vi "Initialize Kinect - Copy.vi"() -> (0 "error out":errorcluster, 3 "Reference Out":T1)   [LabVIEW 2011]
uses:
  <vilib>/vision/Image Controls.llb/IMAQ Image.ctl
  Microsoft.Research.Kinect
panel:
  in  "Buffer Size":i32=1
  in  "error in (no error)":errorcluster
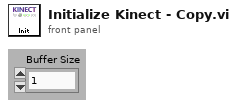
[diagram p1: front panel]
types:
  T1 = cluster{cluster{"queue out":refnum<queue>, "queue out":refnum<queue>}, cluster{"new reference":refnum<k24>, "DepthStream":refnum<k24>, "VideoStream":refnum<k24>, "Event Callback":refnum<k27>, "Event Callback":refnum<k27>}}
  T2 = typedef "IMAQ Image.ctl" = refnum<image>
  T3 = cluster{"queue out":refnum<queue>, "queue out":refnum<queue>}
  T4 = cluster{"new reference":refnum<k24>, "DepthStream":refnum<k24>, "VideoStream":refnum<k24>, refnum<k27>, refnum<k27>}
  T5 = cluster{cluster{"queue out":refnum<queue>, "queue out":refnum<queue>}, cluster{"new reference":refnum<k24>, "DepthStream":refnum<k24>, "VideoStream":refnum<k24>, refnum<k27>, refnum<k27>}}
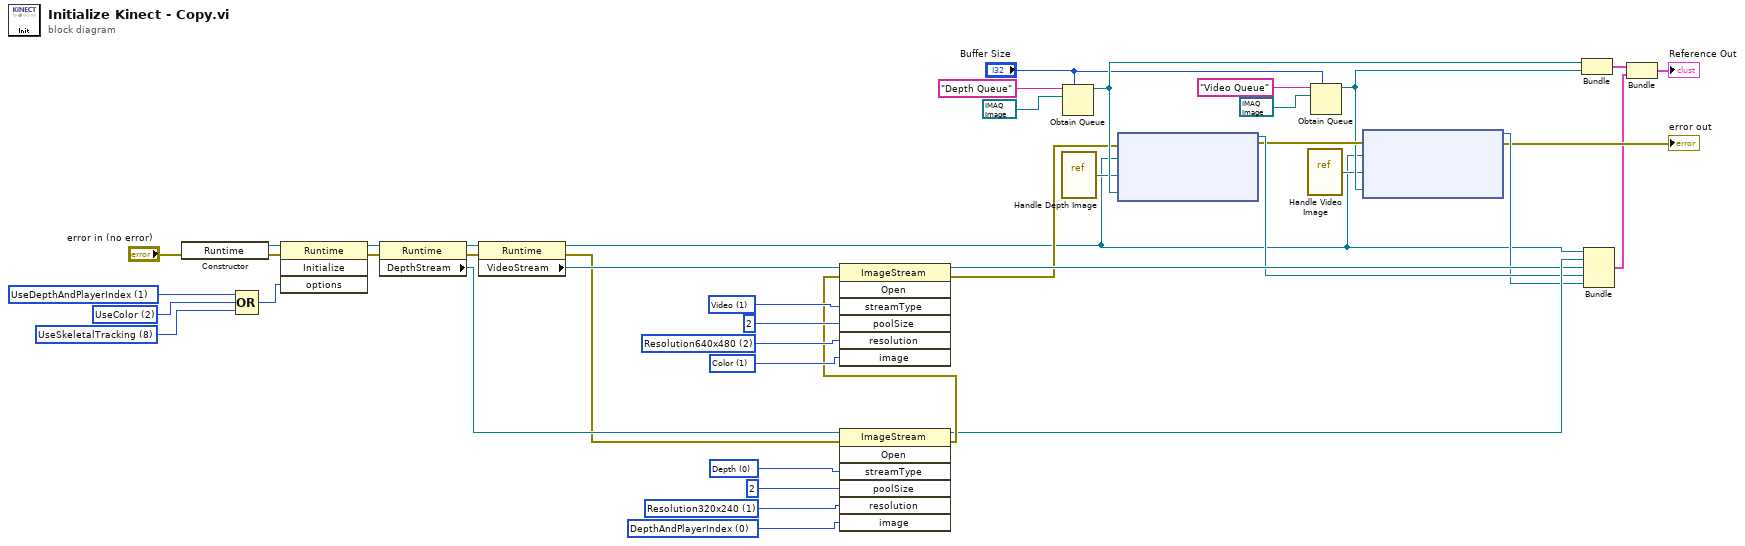
[diagram p0: block diagram]
diagram:
  w25 = 8 items=["UseDepthAndPlayerIndex"=1, "UseColor"=2, "UseSkeletalTracking"=8, "UseDepth"=32] ("options")
  w26 = 2 items=["UseDepthAndPlayerIndex"=1, "UseColor"=2, "UseSkeletalTracking"=8, "UseDepth"=32] ("options")
  w36 = 1 items=["Resolution80x60"=0, "Resolution320x240"=1, "Resolution640x480"=2, "Resolution1280x1024"=3, "Invalid"=-1] ("resolution")
  w27 = 1 items=["UseDepthAndPlayerIndex"=1, "UseColor"=2, "UseSkeletalTracking"=8, "UseDepth"=32] ("options")
  w39 = 0 items=["DepthAndPlayerIndex", "Color", "ColorYuv", "ColorYuvRaw", "Depth", "DepthAndPlayerIndexInColorSpace", "DepthInColorSpace", "ColorInDepthSpace"] ("image")
  w31 = 1 items=["DepthAndPlayerIndex", "Color", "ColorYuv", "ColorYuvRaw", "Depth", "DepthAndPlayerIndexInColorSpace", "DepthInColorSpace", "ColorInDepthSpace"] ("image")
  w32 = 2 items=["Resolution80x60"=0, "Resolution320x240"=1, "Resolution640x480"=2, "Resolution1280x1024"=3, "Invalid"=-1] ("resolution")
  w34 = 1 items=["Depth"=0, "Video"=1, "Invalid"=-1] ("streamType")
  w5 = 0 items=["Depth"=0, "Video"=1, "Invalid"=-1] ("streamType")
  n1 = constructor class="Runtime" ("Constructor Node")(error in="error in (no error)") -> (reference out=w40:refnum<k24>, error out=w38:errorcluster)  [unwired: 2 in, 1 out]
  n2 = Compound Arithmetic op=OR(w27, w26, w25) -> (w37:i32)
  n3 = invoke class="Runtime" method="Initialize"(reference=w40, error in=w38, "options"=w37) -> (reference out=w3:refnum<k24>, error out=w43:errorcluster)  [unwired: 1 in, 2 out]
  n4 = property on="Property Node" class="Runtime"(reference=w3, error in=w43) -> (reference out=w2:refnum<k24>, error out=w30:errorcluster, "DepthStream"=w42:refnum<k24>)
  n5 = property class="Runtime"(reference=w2, error in=w30) -> (reference out=w1:refnum<k24>, error out=w29:errorcluster, "VideoStream"=w35:refnum<k24>)
  n6 = invoke class="ImageStream" method="Open"(reference=w42, error in=w29, "streamType"=w5, "poolSize"=2, "resolution"=w36, "image"=w39) -> (reference out=w24:refnum<k24>, error out=w28:errorcluster)  [unwired: 1 in, 5 out]
  n7 = invoke class="ImageStream" method="Open"(reference=w35, error in=w28, "streamType"=w34, "poolSize"=2, "resolution"=w32, "image"=w31) -> (reference out=w23:refnum<k24>, error out=w4:errorcluster)  [unwired: 1 in, 5 out]
  n8 = vi-ref "Handle Depth Image.vi"() -> ("vi reference"=w11:refnum<vi>)
  n9 = Obtain Queue(max queue size (-1, unlimited)="Buffer Size", name (unnamed)="Depth Queue", element data type=T2 refnum ("New Image")) -> (queue out=w13:refnum<queue>)  [unwired: 2 in, 2 out]
  n10 = node(w4, w1, w11, w13) -> (w22:refnum<k27>, w14:errorcluster)  [unwired: 1 in]
  n11 = vi-ref "Handle Video Image.vi"() -> ("vi reference"=w10:refnum<vi>)
  n12 = Obtain Queue(max queue size (-1, unlimited)="Buffer Size", name (unnamed)="Video Queue", element data type=T2 refnum ("New Image")) -> (queue out=w12:refnum<queue>)  [unwired: 2 in, 2 out]
  n13 = node(w14, w1, w10, w12) -> (w21:refnum<k27>, →"error out":errorcluster)  [unwired: 1 in]
  n14 = Bundle("queue out"=w13, "queue out"=w12) -> (w8:T3)  [unwired: 1 in]
  n15 = Bundle("new reference"=w1, "DepthStream"=w24, "VideoStream"=w23, w22, w21) -> (w7:T4)  [unwired: 1 in]
  n16 = Bundle(w8, w7) -> (→"Reference Out":T5)  [unwired: 1 in]
